vi "Build CAN Interface Name.vi"(11 "CAN Number":i32) -> (3 "CAN Interface Name":string)   [LabVIEW 2025]
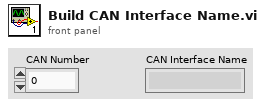
[diagram p1: front panel]
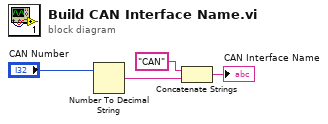
[diagram p0: block diagram]
diagram:
  n1 = Number To Decimal String(number="CAN Number") -> (decimal integer string=w4:string)  [unwired: 1 in]
  n2 = Concatenate Strings("CAN" ("string"), w4) -> (→"CAN Interface Name":string)
